vi "Actor Core.vi"(8 "error in":errorcluster, 11 "Sample PWM Tacho Fans in":refnum<class "Sample PWM Tacho Fans.lvclass">) -> (0 "error out":errorcluster, 3 "Actor out":refnum<class "Actor.lvclass">)   [LabVIEW 2023, in "Sample PWM Tacho Fans.lvlib" / "Sample PWM Tacho Fans.lvclass"]
doc: "(<B>Filename</B>: Actor Framework.lvlib:Actor.lvclass:Actor Core.vi)\n\nReceives messages to the actor, reacts to them, and initiates any error handling that may shut the actor down.\n\nDescendant classes may override this VI to append parallel tasks for the actor to complete while it handles messages. Overrides use the Call Parent Class Method node."
uses:
  Sample PWM Tacho Fans.lvclass
  Sample PWM Tacho Fans.lvclass/Sample PWM Tacho Fans.ctl
  Series/ISeries Actor/ISeries Actor Messages/Stop Tasks Msg/Stop Tasks Msg.lvclass
  Series/ISeries Actor/ISeries Actor Messages/Start Tasks Msg/Start Tasks Msg.lvclass
  <vilib>/ActorFramework/Stop Msg/Stop Msg.lvclass
  Series/ISeries Actor/ISeries Actor Messages/Do Task Msg/Do Task Msg.lvclass
  <vilib>/MGI/Panel Manager/Panel Actor/Panel Actor/Panel Actor.lvclass
  Series/Series Actor/Series Actor/Series Actor.lvclass
  <vilib>/ActorFramework/Actor/Actor.lvclass
panel:
  out "Tacho F2":dbl format="%#_g rpm"
  out "Remote Setpoint F2":dbl format="%#_g %"
  out "Tacho F1":dbl format="%#_g rpm"
  out "Remote Setpoint F1":dbl format="%#_g %"
  in  "Kill Series Button":bool
  in  "Start Button":bool
  in  "Stop Button":bool
  in  "Fan2":dbl(knob) scale=0.0..100.0 scale format="%#_g %"
  in  "Fan1":dbl(knob) scale=0.0..100.0 scale format="%#_g %"
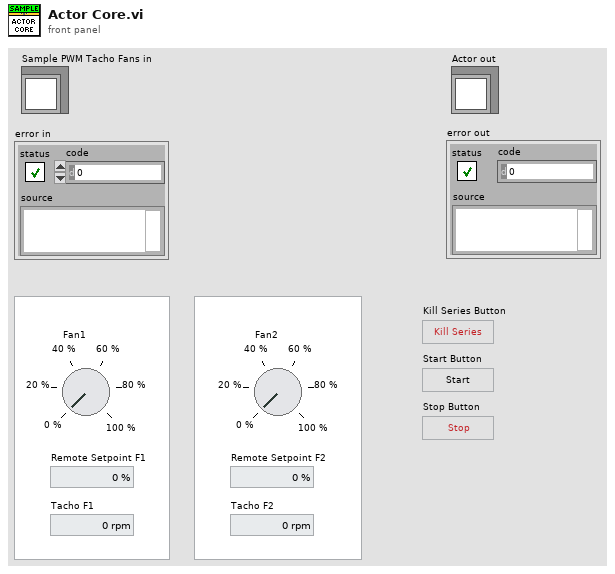
[diagram p1: front panel]
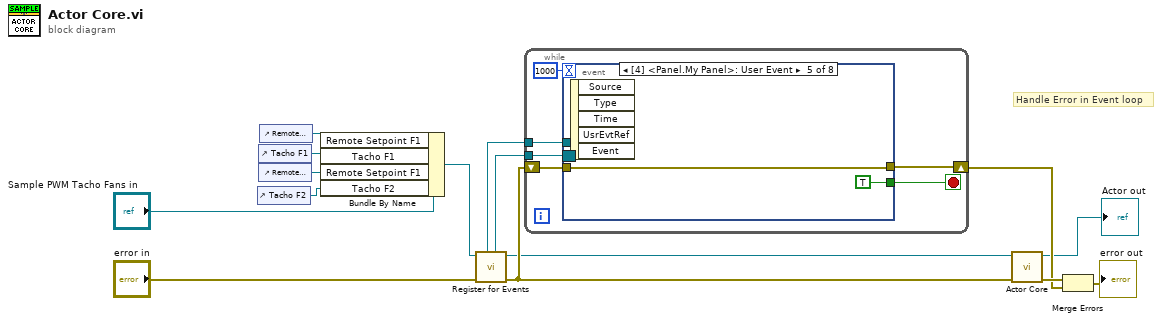
[diagram p0: block diagram]
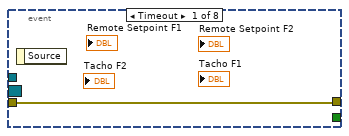
[diagram p2: hidden frame]
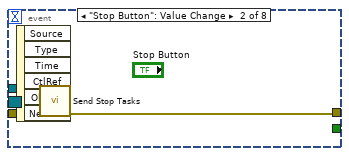
[diagram p3: hidden frame]
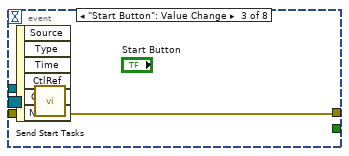
[diagram p4: hidden frame]
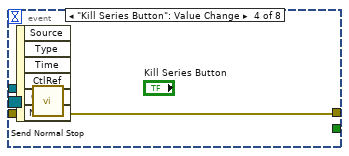
[diagram p5: hidden frame]
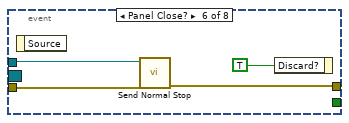
[diagram p6: hidden frame]
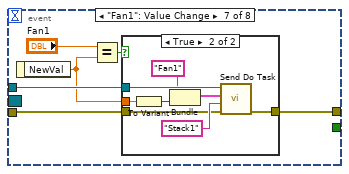
[diagram p7: hidden frame]
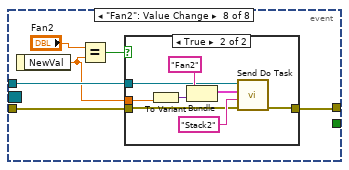
[diagram p9: hidden frame]
diagram:
  # "Handle Error in Event loop"
  n1 = control-ref of="Tacho F2"() -> (w11:refnum<vi>)
  n2 = control-ref of="Tacho F1"() -> (w9:refnum<vi>)
  n3 = control-ref of="Remote Setpoint F2"() -> (w12:refnum<vi>)
  n4 = control-ref of="Remote Setpoint F1"() -> (w10:refnum<vi>)
  n5 = Bundle By Name(cluster="Sample PWM Tacho Fans in", "Remote Setpoint F1"=w10, "Tacho F1"=w9, "Remote Setpoint F1"=w12, "Tacho F2"=w11) -> (w4:refnum<class "Sample PWM Tacho Fans.lvclass">)
  n6 = call <vilib>:"Register for Events.vi"("Error In"="error in", "Panel Actor in"=w4) -> ("Error Out"=w5:errorcluster, "Panel Actor out"=w3:refnum<class "Sample PWM Tacho Fans.lvclass">, "Pnl Actor"=w1:refnum<event-registration>, "Self Enqueuer"=w2:refnum<class "Message Enqueuer.lvclass">)  [unwired: 6 in]
  n7 = while {
    tunnel: w1 -> [w21]
    tunnel: w2 -> [w20]
    shift-right: [w17] -> w13
    shift-left: w5 -> [w19]
    stop <- w16 stop-if-true
    n8 = event shown="[4] <Panel.My Panel>: User Event" {
      selector: w21 -> [_ _ _ _ _ _ _ _]
      dyn-events: _ -> [_ _ _ _ _ _ _ _]
      timeout: 1000 -> [_ _ _ _ _ _ _ _]
      tunnel: w20 -> [_ w24 w27 w30 _ w35 w41 w58]
      tunnel: w19 -> [w22 w25 w28 w31 w32 w36 w42 w57]
      tunnel: [_ _ _ _ TRUE _ _ _] -> w16
      tunnel: [w22 w23 w26 w29 w32 w34 w39 w54] -> w17
      event Timeout {
        n9 = event-data() -> ()  [unwired: 1 in, 1 out]
      }
      event "Stop Button": Value Change {
        n10 = event-data() -> ()  [unwired: 1 in, 6 out]
        n11 = call "Send Stop Tasks.vi"("error in (no error)"=w25, "Message Enqueuer"=w24) -> ("error out"=w23:errorcluster)  [unwired: 8 in, 1 out]
      }
      event "Start Button": Value Change {
        n12 = event-data() -> ()  [unwired: 1 in, 6 out]
        n13 = call "Send Start Tasks.vi"("error in (no error)"=w28, "Message Enqueuer"=w27) -> ("error out"=w26:errorcluster)  [unwired: 8 in, 1 out]
      }
      event "Kill Series Button": Value Change {
        n14 = event-data() -> ()  [unwired: 1 in, 6 out]
        n15 = call <vilib>:"Send Normal Stop.vi"("error in (no error)"=w31, "Message Enqueuer"=w30) -> ("error out"=w29:errorcluster)  [unwired: 9 in]
      }
      event User Event {
        n16 = event-data() -> ()  [unwired: 1 in, 5 out]
      }
      event Panel Close? {
        n17 = event-data() -> ()  [unwired: 1 in, 1 out]
        n18 = call <vilib>:"Send Normal Stop.vi"("error in (no error)"=w36, "Message Enqueuer"=w35) -> ("error out"=w34:errorcluster)  [unwired: 9 in]
        n19 = event-data("Discard?"=TRUE) -> ()  [unwired: 1 in, 1 out]
      }
      event "Fan1": Value Change {
        n20 = event-data() -> ("NewVal"=w40:dbl)  [unwired: 1 in]
        n21 = Equal?(x="Fan1", y=w40) -> (x = y?=w43:bool)
        n22 = case shown="True" w43 {
          tunnel: w41 -> [_ w50]
          tunnel: w42 -> [w44 w49]
          tunnel: w40 -> [_ w45]
          tunnel: [w44 w52] -> w39
          frame False {
          }
          frame True {
            n23 = To Variant(anything=w45) -> (Variant=w46:variant)
            n24 = Bundle("Fan1", "Variant"=w46) -> (w48:cluster{string, "Variant":variant})  [unwired: 1 in]
            n25 = call "Send Do Task.vi"("error in (no error)"=w49, "Task Ident"="Stack1", "Input"=w48, "Message Enqueuer"=w50) -> ("error out"=w52:errorcluster)  [unwired: 6 in, 1 out]
          }
        }
      }
      event "Fan2": Value Change {
        n26 = event-data() -> ("NewVal"=w55:dbl)  [unwired: 1 in]
        n27 = Equal?(x="Fan2", y=w55) -> (x = y?=w56:bool)
        n28 = case shown="True" w56 {
          tunnel: w58 -> [_ w61]
          tunnel: w57 -> [w59 w62]
          tunnel: w55 -> [_ w60]
          tunnel: [w59 w63] -> w54
          frame False {
          }
          frame True {
            n29 = To Variant(anything=w60) -> (Variant=w64:variant)
            n30 = Bundle("Fan2", "Variant"=w64) -> (w66:cluster{string, "Variant":variant})  [unwired: 1 in]
            n31 = call "Send Do Task.vi"("error in (no error)"=w62, "Task Ident"="Stack2", "Input"=w66, "Message Enqueuer"=w61) -> ("error out"=w63:errorcluster)  [unwired: 6 in, 1 out]
          }
        }
      }
    }
  }
  n32 = call-parent "Actor Core.vi"("error in"=w5, "Series Actor in"=w3) -> ("error out"=w15:errorcluster, "Actor out"=→"Actor out":refnum<class "Actor.lvclass">)  [unwired: 8 in]
  n33 = Merge Errors(w15, w13) -> (→"error out":errorcluster)
